vi "Write Digital Sine waveform.vi"(6 "reg0 value":u32, 7 "Waveform name":string, 8 "error in":errorcluster, 9 "Waveform data":u16[](array[numeric]), 11 "Digital session":refnum<k15>) -> (0 "error out":errorcluster, 3 "Digital session out":refnum<k15>)   [LabVIEW 2021, in "Single Tone_DAC.lvlib"]
uses:
  <instrlib>/niDigital/niDigital.llb/niDigital Export Signal.ctl
  <instrlib>/niDigital/niDigital.llb/niDigital Write Source Waveform (Broadcast U32).vi
  <instrlib>/niDigital/niDigital.llb/niDigital Burst Pattern (Burst Only).vi
  Single Tone_DAC.lvlib
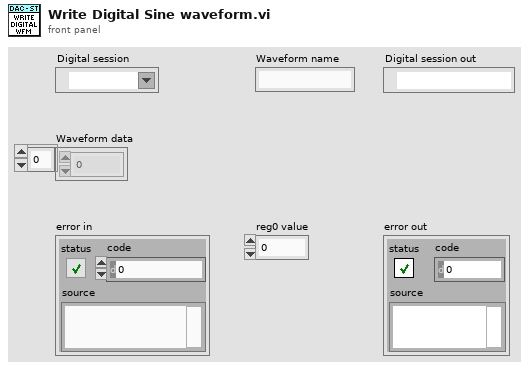
[diagram p1: front panel]
types:
  T1 = typedef "niDigital Export Signal.ctl" = i32
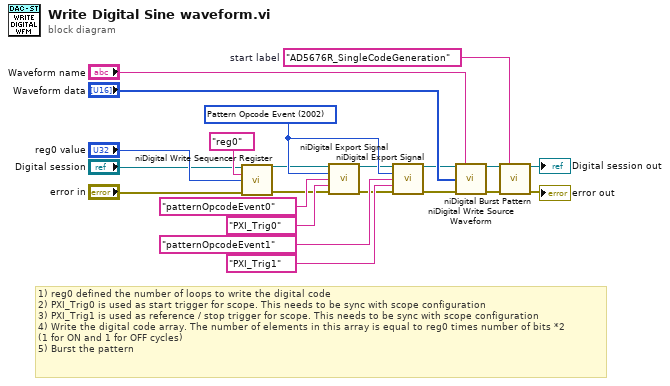
[diagram p0: block diagram]
diagram:
  w21 = "AD5676R_SingleCodeGeneration"  # start label
  w12 = T1 2002 items=["Start Trigger"=2000, "Conditional Jump Trigger"=2001, "Pattern Opcode Event"=2002, "RIO Event"=2004] ("signal")
  # "1) reg0 defined the number of loops to write the digital code\n2) PXI_Trig0 is used as start trigger for scope. This needs to be sync with scope configuration\n3) PXI_Trig1 is used as reference / stop trigger for scope. This needs to be sync with scope configuration\n4) Write the digital code array. The number of elements in this array is equal to reg0 times number of bits *2 \n(1 for ON and 1 for OFF cycles)\n5) Burst the pattern"
  n1 = call <instrlib>:"niDigital Write Sequencer Register.vi"("instrument handle"="Digital session", "sequencer register"="reg0", "value"="reg0 value", "error in"="error in") -> ("instrument handle out"=w6:refnum<k15>, "error out"=w7:errorcluster)  [unwired: 10 in]
  n2 = call <instrlib>:"niDigital Export Signal.vi"("instrument handle"=w6, "signal"=w12, "signal ID"="patternOpcodeEvent0", "output terminal"="PXI_Trig0", "error in"=w7) -> ("instrument handle out"=w10:refnum<k15>, "error out"=w11:errorcluster)  [unwired: 9 in]
  n3 = call <instrlib>:"niDigital Export Signal.vi"("instrument handle"=w10, "signal"=w12, "signal ID"="patternOpcodeEvent1", "output terminal"="PXI_Trig1", "error in"=w11) -> ("instrument handle out"=w15:refnum<k15>, "error out"=w16:errorcluster)  [unwired: 9 in]
  n4 = call-poly <instrlib>:"niDigital Write Source Waveform.vi"("instrument handle"=w15, "waveform name"="Waveform name", "waveform data"="Waveform data", "error in"=w16) -> ("instrument handle out"=w19:refnum<k15>, "error out"=w20:errorcluster)  [unwired: 10 in]
  n5 = call-poly <instrlib>:"niDigital Burst Pattern.vi"("instrument handle"=w19, "start label"=w21, "error in"=w20) -> ("instrument handle out"=→"Digital session out":refnum<k15>, "error out"=→"error out":errorcluster)  [unwired: 11 in]
